vi "Replace Single Wheel in Steering Frame.vi"(5 "x position":dbl, 6 "frame angle (rad)":dbl=nan, 7 "y position":dbl, 8 "error in (no error)":errorcluster, 9 "wheel":refnum<class "NI_Robotics_Wheel.lvclass">, 10 "wheel index":i32, 11 "steering frame in":refnum<class "NI_Robotics_Steering Frame.lvclass">) -> (0 "error out":errorcluster, 1 "found?":bool, 3 "steering frame out":refnum<class "NI_Robotics_Steering Frame.lvclass">)   [LabVIEW 2017, in "NI_Robotics_Steering Frame.lvclass"]
doc: "Replaces wheels in <B>steering frame in</B> with the wheels you specify. You must manually select the polymorphic instance to use."
uses:
  <vilib>/robotics/Steering/Steering Frame/NI_Robotics_Steering Frame.lvclass
  <vilib>/robotics/Steering/Wheel/NI_Robotics_Wheel.lvclass
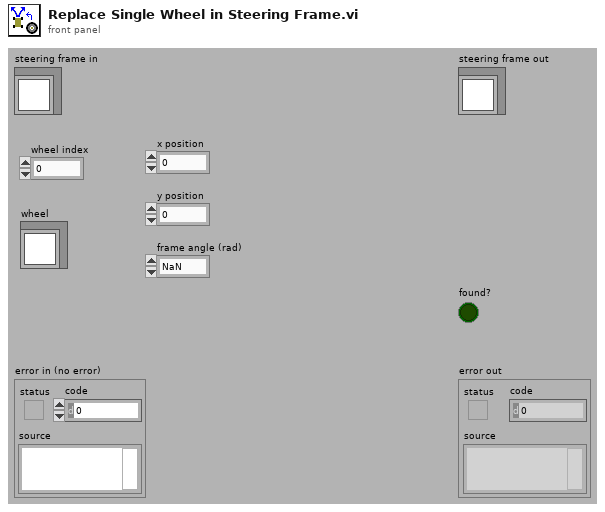
[diagram p1: front panel]
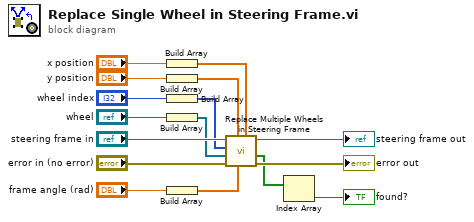
[diagram p0: block diagram]
diagram:
  n1 = Build Array("x position") -> (w2:dbl[])
  n2 = Build Array("y position") -> (w3:dbl[])
  n3 = Build Array("wheel index") -> (w6:i32[])
  n4 = Build Array("wheel") -> (w5:refnum<class "NI_Robotics_Wheel.lvclass">[])
  n5 = Build Array("frame angle (rad)") -> (w1:dbl[])
  n6 = call <vilib>:"Replace Multiple Wheels in Steering Frame.vi"("x positions"=w2, "frame angles (rad)"=w1, "y positions"=w3, "error in (no error)"="error in (no error)", "wheels"=w5, "wheel indexes"=w6, "steering frame in"="steering frame in") -> ("error out"=→"error out":errorcluster, "found?"=w4:bool[], "steering frame out"=→"steering frame out":refnum<class "NI_Robotics_Steering Frame.lvclass">)  [unwired: 2 in]
  n7 = Index Array(array=w4) -> (element=→"found?":bool)  [unwired: 1 in]
